vi "disable_tab.vi"(8 "error in (no error)":errorcluster, 9 "disabled? (F)":bool, 10 "page label":string, 11 "tabs ref":refnum<vi>) -> (0 "error out":errorcluster, 3 "tabs ref (duplicate)":refnum<vi>)   [LabVIEW 2015]
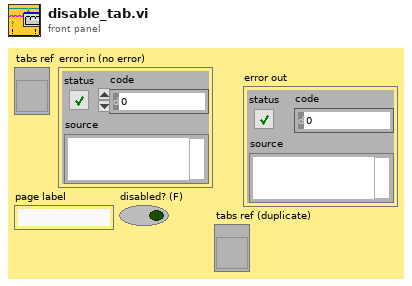
[diagram p1: front panel]
types:
  T1 = enum32{"Page Enabled", "Page Disabled", "Page Disabled & Grayed"}
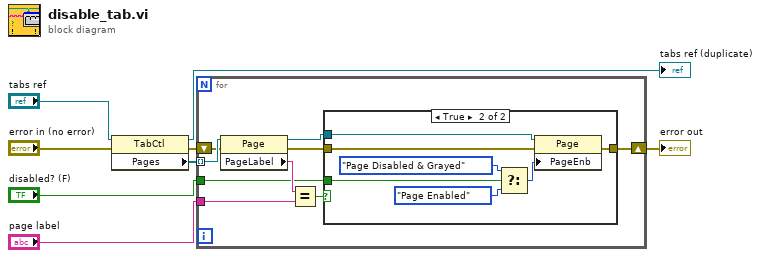
[diagram p0: block diagram]
diagram:
  n1 = property on="Property Node" class="TabCtl"(reference="tabs ref", error in="error in (no error)") -> (reference out=→"tabs ref (duplicate)":refnum<vi>, error out=w7:errorcluster, "Pages"=w8:refnum<vi>[])
  n2 = for {
    tunnel: w8 -> [w17] mode=indexing
    shift-right: [w13] -> w4
    shift-left: w7 -> [w15]
    tunnel: "page label" -> [w11]
    tunnel: "disabled? (F)" -> [w9]
    n3 = property class="Page"(reference=w17, error in=w15) -> (reference out=w16:refnum<vi>, error out=w14:errorcluster, "PageLabel"=w12:string)
    n4 = Equal?(x=w12, y=w11) -> (x = y?=w10:bool)
    n5 = case shown="True" w10 {
      tunnel: w16 -> [_ w25]
      tunnel: w14 -> [w18 w24]
      tunnel: [w18 w23] -> w13
      tunnel: w9 -> [_ w22]
      frame False {
      }
      frame True {
        n6 = Select(t=T1."Page Disabled & Grayed" ("Page Enabled State"), s=w22, f=T1."Page Enabled" ("Page Enabled State")) -> (s? t:f=w19:T1)
        n7 = property class="Page"(reference=w25, error in=w24, "PageEnb"=w19) -> (error out=w23:errorcluster)  [unwired: 1 out]
      }
    }
  }
  "error out" <- w4
